vi "Initialize New.vi"(8 "error in (no error)":errorcluster, 10 "count":i32, 11 "Core Threads Configuration in":refnum<class "Core Threads Configuration.lvclass">) -> (0 "error out":errorcluster, 3 "Core Threads Configuration out":refnum<class "Core Threads Configuration.lvclass">)   [LabVIEW 2017, in "DSF Core.lvlib" / "Core Threads Configuration.lvclass"]
uses:
  Core Threads Configuration.lvclass
  Typedefs/DSF Core Thread Configuration.ctl
  Core Threads Configuration.lvclass/Core Threads Configuration.ctl
  DSF Core.lvlib
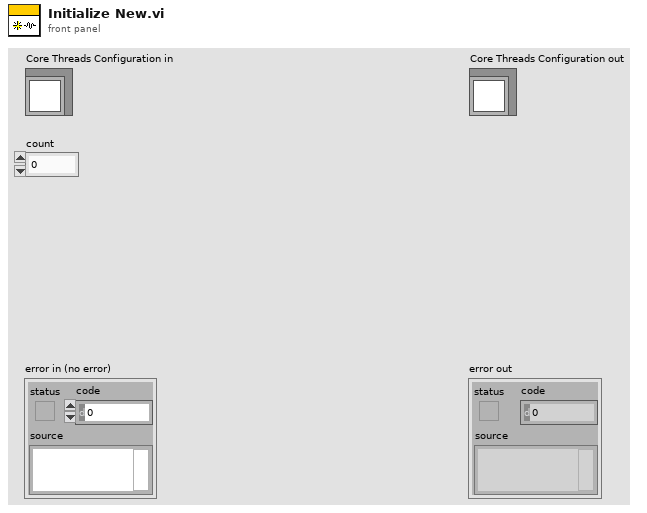
[diagram p1: front panel]
types:
  T1 = typedef "DSF Core.lvlib/DSF Core Thread Configuration.ctl" = cluster{"processor":i32, "priority offset":i16}
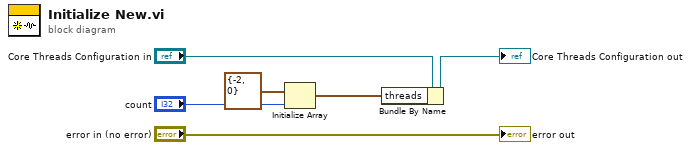
[diagram p0: block diagram]
diagram:
  n1 = Initialize Array(T1 {"processor"=-2, "priority offset"=0} ("thread configurations"), "count") -> (w1:T1[])
  n2 = Bundle By Name(cluster="Core Threads Configuration in", "threads"=w1) -> (→"Core Threads Configuration out":refnum<class "Core Threads Configuration.lvclass">)
  "error out" <- "error in (no error)"
